vi "Create Read Channel.vi"(7 "Name":string, 8 "error in (no error)":errorcluster, 9 "Channel":T2 {"Data Type" format="%.0x"}, 10 "Bitfile Name":string, 11 "Item Ref in":T1 format="%.0x") -> (0 "error out":errorcluster)   [LabVIEW 2018, in "FPGA Addon System Explorer.lvlib"]
uses:
  FPGA Addon System Explorer.lvlib
  Addon Shared/Types/Register Information.ctl
  Addon Shared/Types/Data Type.ctl
  <vilib>/NI Veristand/Custom Device API/Custom Device Item Ref.ctl
  <vilib>/NI Veristand/Custom Device API/Custom Device Channel.ctl
  <vilib>/NI Veristand/Custom Device API/Custom Device Channel Type.ctl
  niveristand-fpga-addon-speciality-io/Source/Types/PWM.Measure.Analog.Result.ctl
  niveristand-fpga-addon-speciality-io/Source/Types/PWM.Measure.Digital.Result.ctl
  niveristand-fpga-addon-speciality-io/Source/Types/Static.Measure.Digital.Measurement.ctl
  niveristand-fpga-addon-speciality-io/Source/Types/QuadratureEncoder.Measure.Digital.Measurement.ctl
  Addon Shared/Types/FG Action.ctl
  Addon Shared/SubVIs/Constants.vi
  <vilib>/NI/NI VeriStand Advanced SysDef API/SysDef API/SysDef.Property.Get.vi
  <vilib>/NI/NI VeriStand Advanced SysDef API/_SubVIs/SysDef.Property.Get.Variant.vi
  <vilib>/NI/NI VeriStand Advanced SysDef API/SysDef API/SysDef.Property.Set.vi
  <vilib>/NI/NI VeriStand Advanced SysDef API/_SubVIs/SysDef.Property.Set.Variant.vi
  niveristand-fpga-addon-speciality-io/Source/Speciality FPGA IO.lvlib
  <vilib>/NI Veristand/Custom Device API/Custom Device API.lvlib
  Addon Shared/FPGA Addon Shared.lvlib
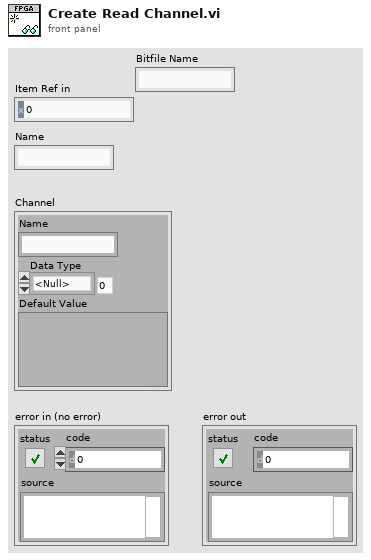
[diagram p1: front panel]
types:
  T1 = typedef "Custom Device API.lvlib/Custom Device Item Ref.ctl" = u64
  T2 = typedef "FPGA Addon Shared.lvlib/Register Information.ctl" = cluster{"Name":string, "Data Type":T3, "Default Value":variant}
  T3 = typedef "FPGA Addon Shared.lvlib/Data Type.ctl" = enum8{"<Null>", "I8", "I16", "I32", "I64", "U8", "U16", "U32", "U64", "SGL", "Boolean", "Analog PWM In Settings", "Analog PWM In", "Digital PWM In Settings", "Digital PWM In", "Digital PWM Out", "Sine Out", "FXP+/-24.5", "FXP+/-16.5", "FXP+/-32.8", "FXP+/-64.32", "FXP+/-16.7", "FXP+/-20.5", "FXP+/-27.5", "FXP+/-32.16", "FXP+16.3", "FXP+18.3", "Digital Static In", "Digital Static Out", "Digital Static In Settings", "Digital WSS Out", "Quad Encoder Settings", "Quad Encoder In", "Group"}
  T4 = typedef "Custom Device API.lvlib/Custom Device Channel.ctl" = cluster{"Type":T5, "Units":string, "Default Value":dbl, "Faultable":bool, "Scalable":bool}
  T5 = typedef "Custom Device API.lvlib/Custom Device Channel Type.ctl" = enum16{"Input", "Output"}
  T6 = typedef "Speciality FPGA IO.lvlib/PWM.Measure.Analog.Result.ctl" = cluster{"FREQ":sgl, "PERIOD":sgl, "DC":sgl, "ACTIVE TIME":sgl, "ACTIVE VOLTAGE":sgl, "INACTIVE VOLTAGE":sgl}
  T7 = typedef "Speciality FPGA IO.lvlib/PWM.Measure.Digital.Result.ctl" = cluster{"FREQ":sgl, "PERIOD":sgl, "DC":sgl, "ACTIVE TIME":sgl}
  T8 = typedef "Speciality FPGA IO.lvlib/Static.Measure.Digital.Measurement.ctl" = cluster{"STATE":bool}
  T9 = typedef "Speciality FPGA IO.lvlib/QuadratureEncoder.Measure.Digital.Measurement.ctl" = cluster{"POSITION":i32}
  T10 = typedef "FPGA Addon Shared.lvlib/FG Action.ctl" = enum8{"GET", "SET"}
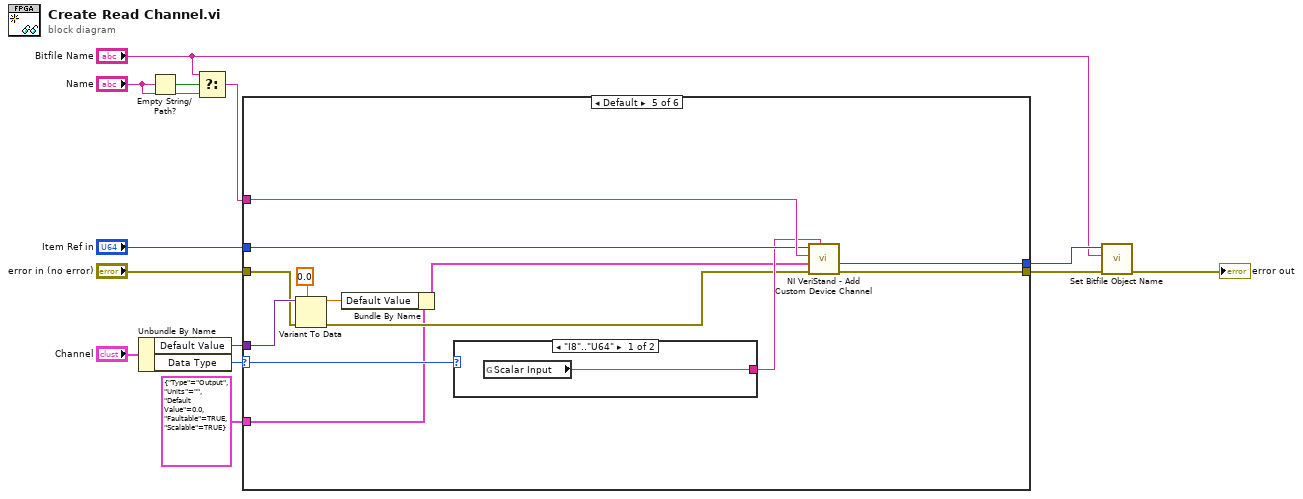
[diagram p0: block diagram]
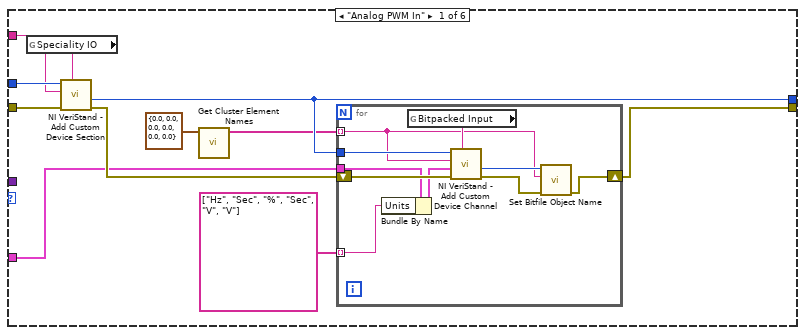
[diagram p2: hidden frame]
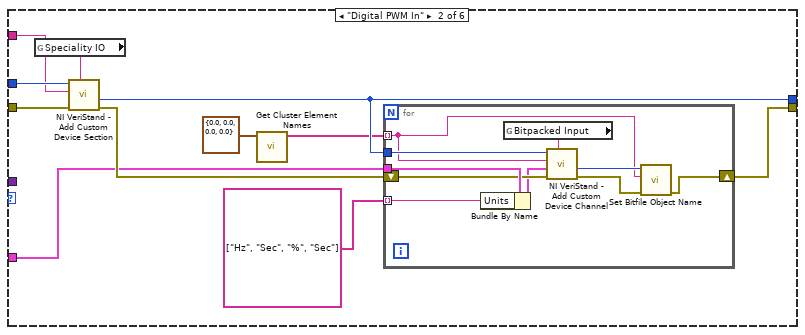
[diagram p3: hidden frame]
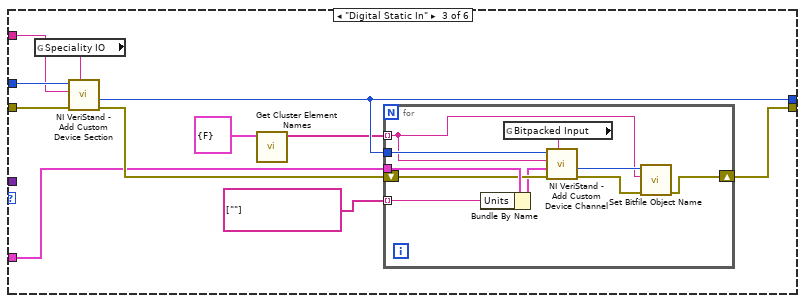
[diagram p4: hidden frame]
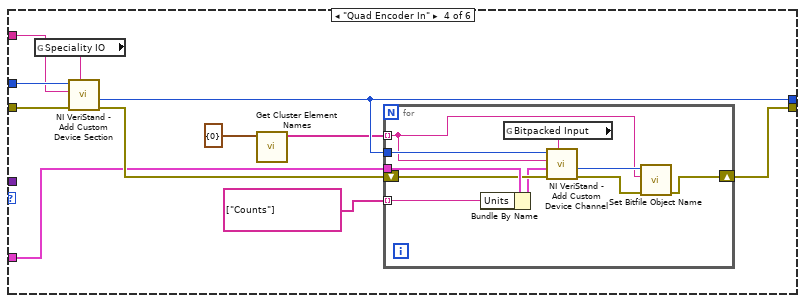
[diagram p5: hidden frame]
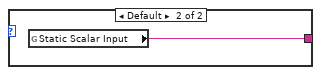
[diagram p6: hidden frame]
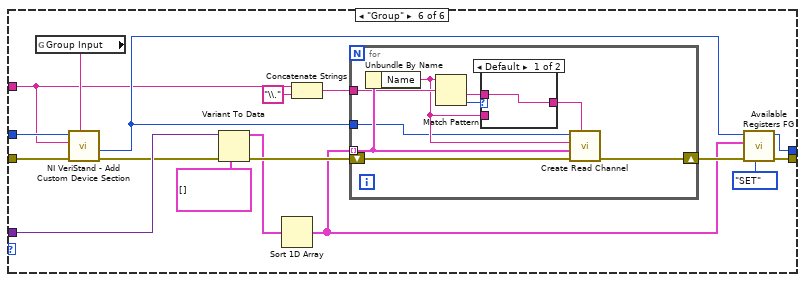
[diagram p7: hidden frame]
diagram:
  n1 = Unbundle By Name("Channel") -> ("Default Value"=w12:variant, "Data Type"=w11:T3)
  n2 = Empty String/Path?(string/path="Name") -> (empty?=w4:bool)
  n3 = Select(t="Bitfile Name", s=w4, f="Name") -> (s? t:f=w1:string)
  n4 = case shown="Default" w11 {
    selector: w11 -> [_ _ _ _ w104 _]
    tunnel: [w20 w41 w62 w83 w110 w121] -> w6
    tunnel: w1 -> [w22 w43 w64 w85 w109 w115]
    tunnel: [w21 w42 w63 w84 w108 w118] -> w7
    tunnel: "error in (no error)" -> [w24 w45 w66 w87 w100 w124]
    tunnel: "Item Ref in" -> [w23 w44 w65 w86 w107 w126]
    tunnel: w12 -> [_ _ _ _ w103 w129]
    tunnel: T4 {"Type"=enum."Output", "Units"="", "Default Value"=0.0, "Faultable"=TRUE, "Scalable"=TRUE} ("Channel") -> [w14 w35 w56 w77 w98 _]
    frame "Analog PWM In" {
      n5 = global read "Constants.vi" "Speciality IO"() -> (w18:string)
      n6 = call <vilib>:"NI VeriStand - Add Custom Device Section.vi"("GUID (Default Section)"=w18, "error in (no error)"=w24, "Section Name"=w22, "Parent Ref in"=w23) -> ("error out"=w15:errorcluster, "Section Ptr"=w21:T1)  [unwired: 4 in, 2 out]
      n7 = call "Get Cluster Element Names.vi"("Cluster"=T6 {"FREQ"=0.0, "PERIOD"=0.0, "DC"=0.0, "ACTIVE TIME"=0.0, "ACTIVE VOLTAGE"=0.0, "INACTIVE VOLTAGE"=0.0} ("Analyzed")) -> ("Channels"=w16:string[])  [unwired: 10 in]
      n8 = for {
        tunnel: w14 -> [w31]
        tunnel: w21 -> [w34]
        shift-right: [w26] -> w20
        shift-left: w15 -> [w33]
        tunnel: string[] ["Hz", "Sec", "%", "Sec", "V", "V"] -> [w29] mode=indexing
        tunnel: w16 -> [w25] mode=indexing
        n9 = Bundle By Name(cluster=w31, "Units"=w29) -> (w30:T4)
        n10 = global read "Constants.vi" "Bitpacked Input"() -> (w32:string)
        n11 = call <vilib>:"NI VeriStand - Add Custom Device Channel.vi"("GUID (Default Channel)"=w32, "error in (no error)"=w33, "Channel"=w30, "Channel Name"=w25, "Parent Ref in"=w34) -> ("error out"=w27:errorcluster, "Channel Ref"=w28:T1)  [unwired: 3 in, 2 out]
        n12 = call "Set Bitfile Object Name.vi"("error in (no error)"=w27, "Name"=w25, "Channel Ref"=w28) -> ("error out"=w26:errorcluster)  [unwired: 8 in]
      }
    }
    frame "Digital PWM In" {
      n13 = global read "Constants.vi" "Speciality IO"() -> (w39:string)
      n14 = call <vilib>:"NI VeriStand - Add Custom Device Section.vi"("GUID (Default Section)"=w39, "error in (no error)"=w45, "Section Name"=w43, "Parent Ref in"=w44) -> ("error out"=w36:errorcluster, "Section Ptr"=w42:T1)  [unwired: 4 in, 2 out]
      n15 = call "Get Cluster Element Names.vi"("Cluster"=T7 {"FREQ"=0.0, "PERIOD"=0.0, "DC"=0.0, "ACTIVE TIME"=0.0} ("Analyzed")) -> ("Channels"=w37:string[])  [unwired: 10 in]
      n16 = for {
        tunnel: w35 -> [w55]
        tunnel: w42 -> [w54]
        shift-right: [w46] -> w41
        shift-left: w36 -> [w53]
        tunnel: string[] ["Hz", "Sec", "%", "Sec"] -> [w50] mode=indexing
        tunnel: w37 -> [w48] mode=indexing
        n17 = Bundle By Name(cluster=w55, "Units"=w50) -> (w51:T4)
        n18 = global read "Constants.vi" "Bitpacked Input"() -> (w52:string)
        n19 = call <vilib>:"NI VeriStand - Add Custom Device Channel.vi"("GUID (Default Channel)"=w52, "error in (no error)"=w53, "Channel"=w51, "Channel Name"=w48, "Parent Ref in"=w54) -> ("error out"=w47:errorcluster, "Channel Ref"=w49:T1)  [unwired: 3 in, 2 out]
        n20 = call "Set Bitfile Object Name.vi"("error in (no error)"=w47, "Name"=w48, "Channel Ref"=w49) -> ("error out"=w46:errorcluster)  [unwired: 8 in]
      }
    }
    frame "Digital Static In" {
      n21 = global read "Constants.vi" "Speciality IO"() -> (w60:string)
      n22 = call <vilib>:"NI VeriStand - Add Custom Device Section.vi"("GUID (Default Section)"=w60, "error in (no error)"=w66, "Section Name"=w64, "Parent Ref in"=w65) -> ("error out"=w57:errorcluster, "Section Ptr"=w63:T1)  [unwired: 4 in, 2 out]
      n23 = call "Get Cluster Element Names.vi"("Cluster"=T8 {"STATE"=FALSE} ("Analyzed")) -> ("Channels"=w58:string[])  [unwired: 10 in]
      n24 = for {
        tunnel: w56 -> [w76]
        tunnel: w63 -> [w75]
        shift-right: [w67] -> w62
        shift-left: w57 -> [w74]
        tunnel: string[] [""] -> [w71] mode=indexing
        tunnel: w58 -> [w69] mode=indexing
        n25 = Bundle By Name(cluster=w76, "Units"=w71) -> (w72:T4)
        n26 = global read "Constants.vi" "Bitpacked Input"() -> (w73:string)
        n27 = call <vilib>:"NI VeriStand - Add Custom Device Channel.vi"("GUID (Default Channel)"=w73, "error in (no error)"=w74, "Channel"=w72, "Channel Name"=w69, "Parent Ref in"=w75) -> ("error out"=w68:errorcluster, "Channel Ref"=w70:T1)  [unwired: 3 in, 2 out]
        n28 = call "Set Bitfile Object Name.vi"("error in (no error)"=w68, "Name"=w69, "Channel Ref"=w70) -> ("error out"=w67:errorcluster)  [unwired: 8 in]
      }
    }
    frame "Quad Encoder In" {
      n29 = global read "Constants.vi" "Speciality IO"() -> (w81:string)
      n30 = call <vilib>:"NI VeriStand - Add Custom Device Section.vi"("GUID (Default Section)"=w81, "error in (no error)"=w87, "Section Name"=w85, "Parent Ref in"=w86) -> ("error out"=w78:errorcluster, "Section Ptr"=w84:T1)  [unwired: 4 in, 2 out]
      n31 = call "Get Cluster Element Names.vi"("Cluster"=T9 {"POSITION"=0} ("Analyzed")) -> ("Channels"=w79:string[])  [unwired: 10 in]
      n32 = for {
        tunnel: w77 -> [w97]
        tunnel: w84 -> [w96]
        shift-right: [w88] -> w83
        shift-left: w78 -> [w95]
        tunnel: string[] ["Counts"] -> [w92] mode=indexing
        tunnel: w79 -> [w90] mode=indexing
        n33 = Bundle By Name(cluster=w97, "Units"=w92) -> (w93:T4)
        n34 = global read "Constants.vi" "Bitpacked Input"() -> (w94:string)
        n35 = call <vilib>:"NI VeriStand - Add Custom Device Channel.vi"("GUID (Default Channel)"=w94, "error in (no error)"=w95, "Channel"=w93, "Channel Name"=w90, "Parent Ref in"=w96) -> ("error out"=w89:errorcluster, "Channel Ref"=w91:T1)  [unwired: 3 in, 2 out]
        n36 = call "Set Bitfile Object Name.vi"("error in (no error)"=w89, "Name"=w90, "Channel Ref"=w91) -> ("error out"=w88:errorcluster)  [unwired: 8 in]
      }
    }
    frame Default {
      n37 = Variant To Data(error in=w100, type=0.0, Variant=w103) -> (data=w101:dbl, error out=w99:errorcluster)
      n38 = Bundle By Name(cluster=w98, "Default Value"=w101) -> (w105:T4)
      n39 = case shown="\"I8\"..\"U64\"" w104 {
        tunnel: [w111 w112] -> w106
        frame "I8".."U64" {
          n40 = global read "Constants.vi" "Scalar Input"() -> (w111:string)
        }
        frame Default {
          n41 = global read "Constants.vi" "Static Scalar Input"() -> (w112:string)
        }
      }
      n42 = call <vilib>:"NI VeriStand - Add Custom Device Channel.vi"("GUID (Default Channel)"=w106, "error in (no error)"=w99, "Channel"=w105, "Channel Name"=w109, "Parent Ref in"=w107) -> ("error out"=w110:errorcluster, "Channel Ref"=w108:T1)  [unwired: 3 in, 2 out]
    }
    frame "Group" {
      n43 = global read "Constants.vi" "Group Input"() -> (w117:string)
      n44 = call <vilib>:"NI VeriStand - Add Custom Device Section.vi"("GUID (Default Section)"=w117, "error in (no error)"=w124, "Section Name"=w115, "Parent Ref in"=w126) -> ("error out"=w125:errorcluster, "Section Ptr"=w119:T1)  [unwired: 4 in, 2 out]
      n45 = Variant To Data(error in=w125, type=T2[] [], Variant=w129) -> (data=w120:T2[], error out=w127:errorcluster)
      n46 = Sort 1D Array(array=w120) -> (sorted array=w116:T2[])
      n47 = Concatenate Strings(w115, "\\.") -> (w113:string)
      n48 = for {
        tunnel: w116 -> [w137] mode=indexing
        shift-right: [w136] -> w122
        shift-left: w127 -> [w138]
        tunnel: w119 -> [w130]
        tunnel: w113 -> [w135]
        n49 = Unbundle By Name(w137) -> ("Name"=w132:string)
        n50 = Match Pattern(string=w132, regular expression=w135) -> (after substring=w133:string, offset past match=w134:i32)  [unwired: 1 in, 2 out]
        n51 = case shown="Default" w134 {
          tunnel: [w139 w140] -> w131
          tunnel: w133 -> [w139 _]
          tunnel: w132 -> [_ w140]
          frame Default {
          }
          frame -1 {
          }
        }
        n52 = call "Create Read Channel.vi"("Name"=w131, "error in (no error)"=w138, "Channel"=w137, "Bitfile Name"=w132, "Item Ref in"=w130) -> ("error out"=w136:errorcluster)  [unwired: 6 in]
      }
      n53 = call "Available Registers FG.vi"("Action"=FG_Action."SET", "error in (no error)"=w122, "Available Registers"=w116, "Item Ref"=w119) -> ("error out"=w121:errorcluster, "Item Ref out"=w118:T1)  [unwired: 5 in, 1 out]
    }
  }
  n54 = call "Set Bitfile Object Name.vi"("error in (no error)"=w6, "Name"="Bitfile Name", "Channel Ref"=w7) -> ("error out"=→"error out":errorcluster)  [unwired: 8 in]
